vi "GetVariableValue.vi"(0 "error in":errorcluster, 5 "Telnet":refnum<k24>, 9 "name":string, 11 "program":string) -> (4 "error out":errorcluster, 6 "KclCommand":string, 8 "Succeed":bool, 10 "ErrorText":string, 15 "RawValue":string)   [LabVIEW 2023, in "UnderAutomation.Fanuc.lvlib"]
uses:
  UnderAutomation.Fanuc.lvlib
  C:/Users/fg/Documents/Fanuc.vi/LabVIEW_2024/UnderAutomation.Fanuc/lib/UnderAutomation.Fanuc.dll
  LabVIEW_2024/UnderAutomation.Fanuc/lib/UnderAutomation.Fanuc.dll
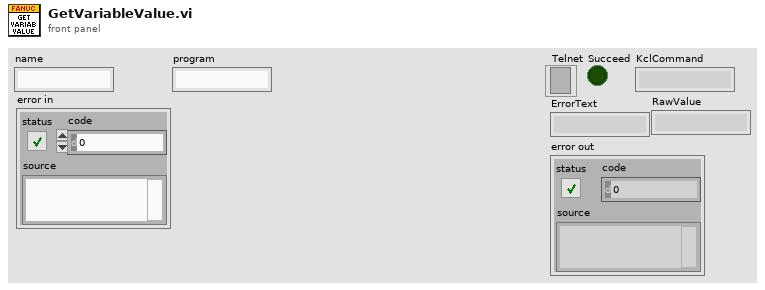
[diagram p1: front panel]
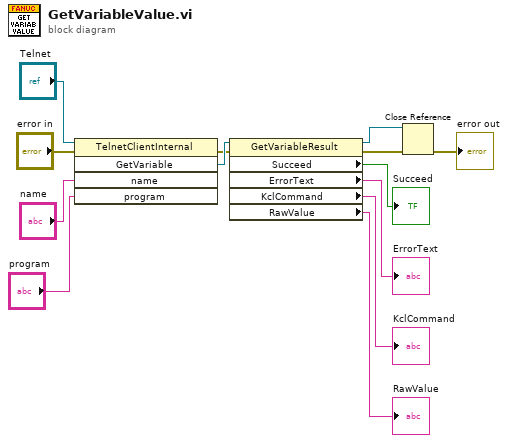
[diagram p0: block diagram]
diagram:
  n1 = invoke class="TelnetClientInternal" method="GetVariable"(reference="Telnet", error in="error in", "name"="name", "program"="program") -> (error out=w8:errorcluster, "GetVariable"=w11:refnum<k24>)  [unwired: 1 in, 3 out]
  n2 = property class="GetVariableResult"(reference=w11, error in=w8) -> (reference out=w4:refnum<k24>, error out=w5:errorcluster, "Succeed"=→"Succeed":bool, "ErrorText"=→"ErrorText":string, "KclCommand"=→"KclCommand":string, "RawValue"=→"RawValue":string)
  n3 = Close Reference(reference=w4, error in (no error)=w5) -> (error out=→"error out":errorcluster)
